vi "NI GetVert.vi"(4 "error in":errorcluster, 6 "Channel (0)":i32, 7 "InstrumentID":refnum<k15>) -> (0 "error out":errorcluster, 1 "index of element":i32, 2 "V scale":T1 {"Coupling" items=["DC 1 MOhm", "AC 1 MOhm", "DC 50 Ohm", "AC 50 OHM"]; "Offset" format="%.2f"}, 3 "Instrument ID out":refnum<k15>)   [LabVIEW 2022 SP3]
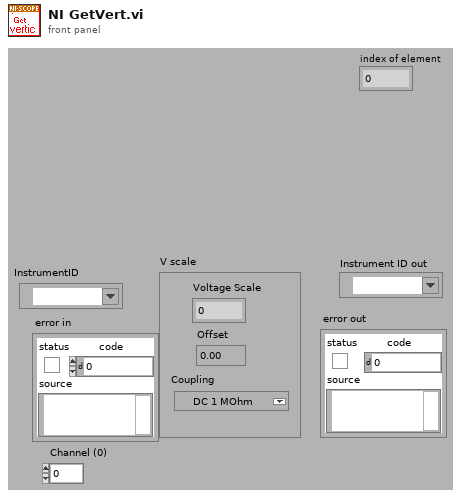
[diagram p1: front panel]
types:
  T1 = cluster{"Voltage Scale":dbl, "Offset":dbl, "Coupling":u16}
  T2 = cluster{"Vertical Range":dbl, "Vertical Offset":dbl, "Coupling":u16}
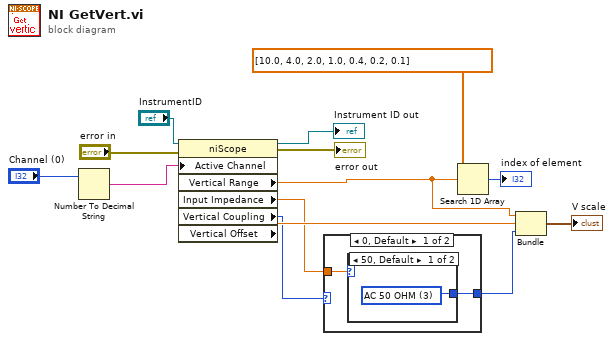
[diagram p0: block diagram]
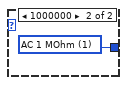
[diagram p2: hidden frame]
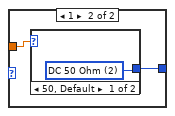
[diagram p3: hidden frame]
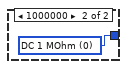
[diagram p4: hidden frame]
diagram:
  n1 = Number To Decimal String(number="Channel (0)") -> (decimal integer string=w3:string)  [unwired: 1 out]
  n2 = property class="niScope"(reference="InstrumentID", error in="error in", "Active Channel"=w3) -> (reference out=→"Instrument ID out":refnum<k15>, error out=→"error out":errorcluster, "Vertical Range"=w2:dbl, "Input Impedance"=w7:dbl, "Vertical Coupling"=w8:i32, "Vertical Offset"=w13:dbl)
  n3 = case shown="0, Default" w8 {
    tunnel: w7 -> [w16 w20]
    tunnel: [w15 w19] -> w6
    frame 0, Default {
      n4 = case shown="50, Default" w16 {
        tunnel: [w17 w18] -> w15
        frame 50, Default {
          w17 = u16 3 items=["DC 1 MOhm", "AC 1 MOhm", "DC 50 Ohm", "AC 50 OHM"] ("Coupling")
        }
        frame 1000000 {
          w18 = u16 1 items=["DC 1 MOhm", "AC 1 MOhm", "DC 50 Ohm", "AC 50 OHM"] ("Coupling")
        }
      }
    }
    frame 1 {
      n5 = case shown="50, Default" w20 {
        tunnel: [w21 w22] -> w19
        frame 50, Default {
          w21 = u16 2 items=["DC 1 MOhm", "AC 1 MOhm", "DC 50 Ohm", "AC 50 OHM"] ("Coupling")
        }
        frame 1000000 {
          w22 = u16 0 items=["DC 1 MOhm", "AC 1 MOhm", "DC 50 Ohm", "AC 50 OHM"] ("Coupling")
        }
      }
    }
  }
  n6 = Search 1D Array(1D array=dbl[] [10.0, 4.0, 2.0, 1.0, 0.4, 0.2, 0.1], element=w2) -> (index of element=→"index of element":i32)  [unwired: 1 out]
  n7 = Bundle("Vertical Range"=w2, "Vertical Offset"=w13, "Coupling"=w6) -> (→"V scale":T2)  [unwired: 1 out]
